vi "write TBM configuration.vi"(8 "error in":errorcluster, 10 "configuration":refnum<class "TBM configuration.lvclass">, 11 "cRIO in":refnum<class "PLTarget cRIO.lvclass">) -> (0 "error out":errorcluster, 3 "cRIO out":refnum<class "PLTarget cRIO.lvclass">)   [LabVIEW 2013, in "PLTarget cRIO.lvclass"]
uses:
  PLTarget cRIO.lvclass
  <vilib>/NI/Tag Bus Module Framework/root configuration/TBM configuration.lvclass
  Framework Configuration Classes/target configuration/PL_Target Configuration.lvclass
  PLTarget cRIO.lvclass/PLTarget cRIO.ctl
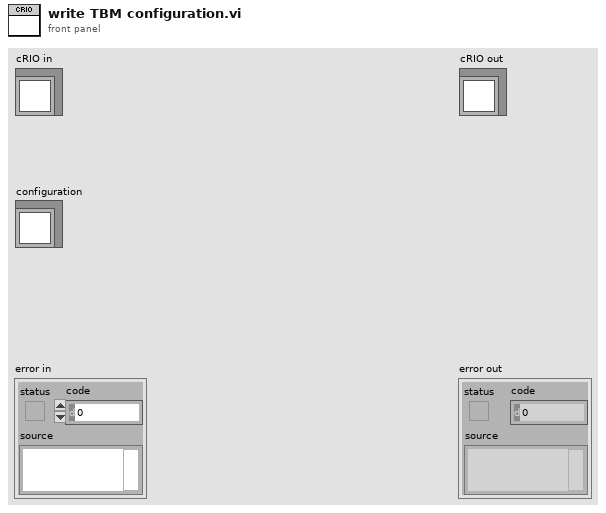
[diagram p1: front panel]
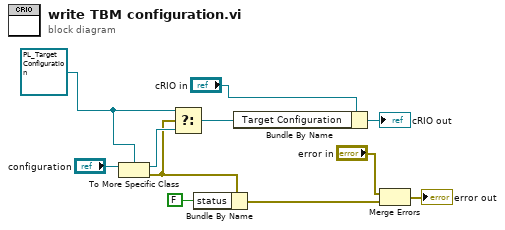
[diagram p0: block diagram]
diagram:
  w2 = refnum<class "PL_Target Configuration.lvclass"> refnum ("Target Configuration")
  n1 = To More Specific Class(target class=w2, reference="configuration") -> (specific class reference=w11:refnum<class "PL_Target Configuration.lvclass">, error out=w10:errorcluster)  [unwired: 1 in]
  n2 = Select(t=w2, s=w10, f=w11) -> (s? t:f=w1:refnum<class "PL_Target Configuration.lvclass">)
  n3 = Bundle By Name(cluster=w10, "status"=FALSE) -> (w8:errorcluster)
  n4 = Bundle By Name(cluster="cRIO in", "Target Configuration"=w1) -> (→"cRIO out":refnum<class "PLTarget cRIO.lvclass">)
  n5 = Merge Errors("error in", w8) -> (→"error out":errorcluster)
